vi "Launch Root DAQmx Actor.vi"(4 "Debug Alias":string, 6 "Open Actor Core front panel? (F)":bool, 7 "DAQmx Task":refnum<k21>, 8 "error in (no error)":errorcluster, 10 "DAQmx Actor":refnum<class "DAQmx Actor.lvclass">) -> (0 "error out":errorcluster, 2 "Actor's Enqueuer":refnum<class "Message Enqueuer.lvclass">)   [LabVIEW 2024]
uses:
  DAQmx Actor.lvclass
  <vilib>/ActorFramework/Message Enqueuer/Message Enqueuer.lvclass
  DAQmx Actor.lvclass/DAQmx Actor.ctl
  <vilib>/ActorFramework/Actor/Actor.lvclass
  C:/Program Files (x86)/National Instruments/LabVIEW 2024/vi.lib/ActorFramework/Actor/Actor.lvclass
  C:/Users/ottoa/OneDrive/Desktop/working copies/DAQmxActor/src/DAQmx Actor/DAQmx Actor/DAQmx Actor.lvclass
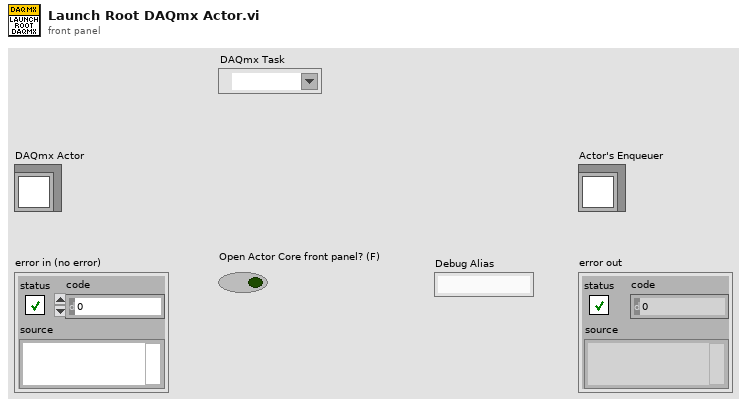
[diagram p1: front panel]
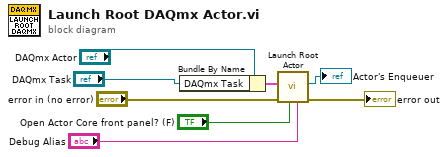
[diagram p0: block diagram]
diagram:
  n1 = Bundle By Name(cluster="DAQmx Actor", "DAQmx Task"="DAQmx Task") -> (w7:cluster{})
  n2 = call <vilib>:"Launch Root Actor.vi"("Debug Alias"="Debug Alias", "Open Actor Core front panel? (F)"="Open Actor Core front panel? (F)", "error in (no error)"="error in (no error)", "Actor"=w7) -> ("error out"=→"error out":errorcluster, "Actor's Enqueuer"=→"Actor's Enqueuer":refnum<class "Message Enqueuer.lvclass">)  [unwired: 6 in]
